vi "Calculate capacity from CV.vi"(2 "t values":dbl[](array[numeric]), 3 "I values":dbl[](array[numeric])) -> (0 "Capacity values":dbl[](array[numeric]))   [LabVIEW 2015]
uses:
  <vilib>/Analysis/NI_AALPro.lvlib
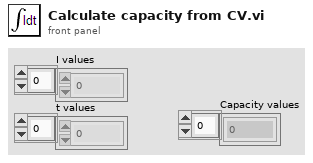
[diagram p1: front panel]
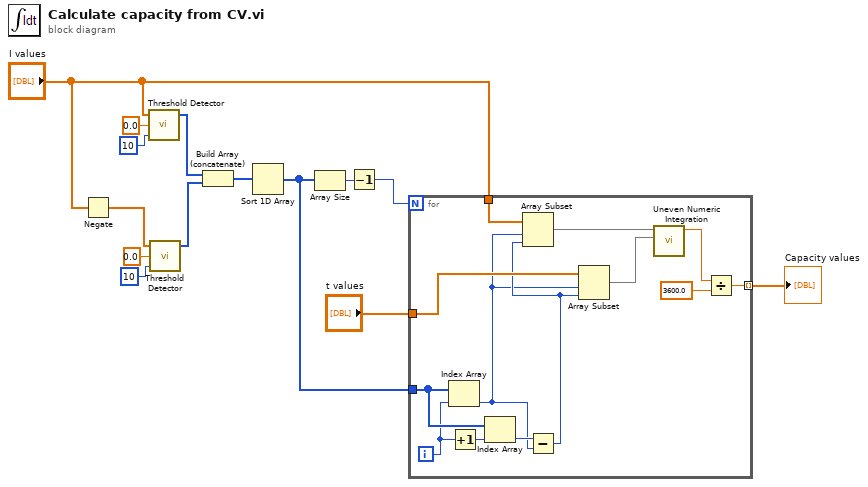
[diagram p0: block diagram]
diagram:
  n1 = Negate(x="I values") -> (-x=w10:dbl[])
  n2 = call <vilib>:"Threshold Detector.vi"("width"=10, "threshold"=0.0, "X"="I values") -> ("Indices"=w9:i32[])  [unwired: 2 out]
  n3 = call <vilib>:"Threshold Detector.vi"("width"=10, "threshold"=0.0, "X"=w10) -> ("Indices"=w8:i32[])  [unwired: 2 out]
  n4 = Build Array (concatenate)(w9, w8) -> (w7:i32[])
  n5 = Sort 1D Array(array=w7) -> (sorted array=w4:i32[])
  n6 = Array Size(array=w4) -> (size(s)=w6:i32)
  n7 = Decrement(x=w6) -> (x-1=w5:i32)
  n8 = for {
    N: w5 -> [_]
    tunnel: w4 -> [w27]
    tunnel: "I values" -> [w24]
    tunnel: "t values" -> [w22]
    tunnel: [w15] -> w1 mode=indexing
    i -> [w25]
    n9 = Index Array(array=w27, index=w25) -> (element=w20:i32)
    n10 = Increment(x=w25) -> (x+1=w26:i32)
    n11 = Index Array(array=w27, index=w26) -> (element=w23:i32)
    n12 = Subtract(x=w23, y=w20) -> (x-y=w21:i32)
    n13 = Array Subset(array=w24, index=w20, length=w21) -> (w18:dbl[])
    n14 = Array Subset(array=w22, index=w20, length=w21) -> (w19:dbl[])
    n15 = call <vilib>:"Uneven Numeric Integration.vi"("T"=w19, "X"=w18) -> ("result"=w16:dbl)  [unwired: 8 in, 1 out]
    n16 = Divide(x=w16, y=3600.0) -> (x/y=w15:dbl)
  }
  "Capacity values" <- w1
